vi "geve-msg-macro-acquire.vi"(8 "error in (no error)":errorcluster, 11 "Runtime Data":T1) -> (0 "error out":errorcluster, 3 "Runtime Data out":T1)   [LabVIEW 2018]
doc: "enqueue sequence for aqn :\nupdate title bar\nread serial data\nparse data\nupdate numerical indicators \nupdate graphs"
uses:
  geve-runtime_data_cluster.ctl
  geve-monitoring_data_cluster.ctl
  geve-serial_config_cluster.ctl
  geve-com_ref_cluster.ctl
  geve-message_cluster.ctl
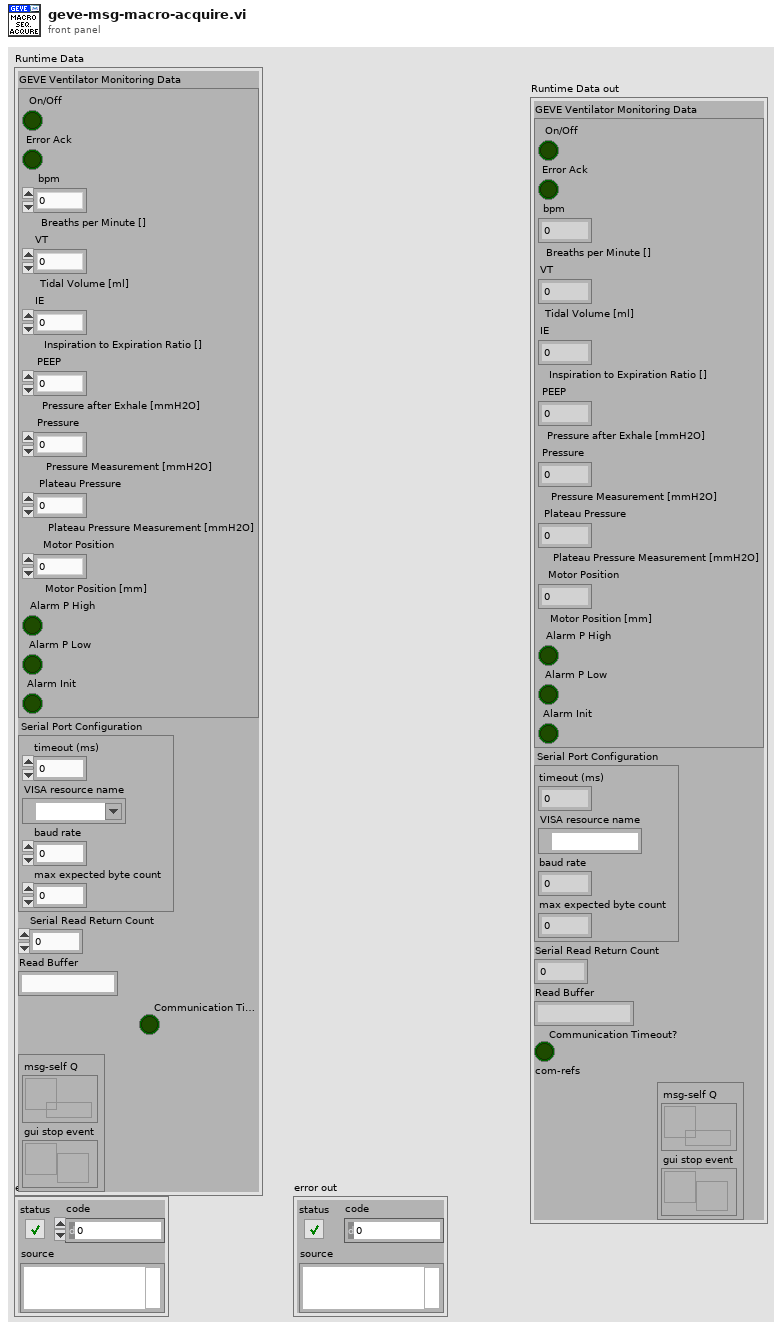
[diagram p1: front panel]
types:
  T1 = typedef "geve-runtime_data_cluster.ctl" = cluster{"GEVE Ventilator Monitoring Data":T2, "Serial Port Configuration":T3, "Serial Read Return Count":u32, "Read Buffer":string, "Communication Timeout?":bool, "com-refs":T4}
  T2 = typedef "geve-monitoring_data_cluster.ctl" = cluster{"On/Off":bool, "Error Ack":bool, "bpm":dbl, "VT":dbl, "IE":dbl, "PEEP":dbl, "Pressure":dbl, "Plateau Pressure":dbl, "Motor Position":dbl, "Alarm P High":bool, "Alarm P Low":bool, "Alarm Init":bool}
  T3 = typedef "geve-serial_config_cluster.ctl" = cluster{"timeout (ms)":u32, "VISA resource name":refnum<visa-resource-name>, "baud rate":u32, "max expected byte count":u32}
  T4 = typedef "geve-com_ref_cluster.ctl" = cluster{"msg-self Q":refnum<queue>, "gui stop event":refnum<user-event>}
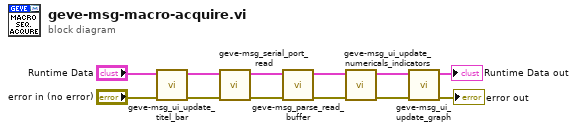
[diagram p0: block diagram]
diagram:
  n1 = call "geve-msg_ui_update_titel_bar.vi"("error in (no error)"="error in (no error)", "Runtime Data"="Runtime Data") -> ("error out"=w7:errorcluster, "Runtime Data out"=w6:T1)  [unwired: 8 in]
  n2 = call "geve-msg_serial_port_read.vi"("error in (no error)"=w7, "Runtime Data"=w6) -> ("error out"=w12:errorcluster, "Runtime Data out"=w5:T1)  [unwired: 8 in]
  n3 = call "geve-msg_parse_read_buffer.vi"("error in (no error)"=w12, "Runtime Data"=w5) -> ("error out"=w11:errorcluster, "Runtime Data out"=w4:T1)  [unwired: 8 in]
  n4 = call "geve-msg_ui_update_numericals_indicators.vi"("error in (no error)"=w11, "Runtime Data"=w4) -> ("error out"=w10:errorcluster, "Runtime Data out"=w2:T1)  [unwired: 8 in]
  n5 = call "geve-msg_ui_update_graph.vi"("error in (no error)"=w10, "Runtime Data"=w2) -> ("error out"=→"error out":errorcluster, "Runtime Data out"=→"Runtime Data out":T1)  [unwired: 8 in]
